vi "DCMotorControl_v2.vi"() -> ()   [LabVIEW 2019]
uses:
  <vilib>/myRIO/Common/Instrument Driver Framework/myRIO v1.0/Encoder/typedefs/Encoder Signal Mode.ctl
  <vilib>/myRIO/Instrument Drivers/Onboard IO/Encoder/typedefs/Encoder Reference.ctl
  <vilib>/myRIO/Common/Instrument Driver Framework/Utilities/typedefs/myRIO Generic Hardware Reference.ctl
  <vilib>/myRIO/Common/Instrument Driver Framework/Utilities/typedefs/Hardware Version Enum.ctl
  <vilib>/myRIO/Common/Instrument Driver Framework/Utilities/typedefs/myRIO v1.0 Reference.ctl
  <vilib>/myRIO/Common/Instrument Driver Framework/Utilities/typedefs/Generic FPGA Reference.ctl
  <vilib>/myRIO/Common/Instrument Driver Framework/myRIO v1.0/Encoder/typedefs/Encoder Channels Enum.ctl
  <vilib>/myRIO/Common/Instrument Driver Framework/myRIO v1.0/Encoder/typedefs/Encoder Configuration v1.0.ctl
  <vilib>/userDefined/High Color/nirio_resource_hc.ctl
  <vilib>/Platform/TimedLoop/XDataNode/timing_clust.ctl
  <vilib>/Platform/TimedLoop/XDataNode/nitl_modes.ctl
  <vilib>/Platform/TimedLoop/XDataNode/wakeup.ctl
  <vilib>/myRIO/Instrument Drivers/Onboard IO/DIO/typedefs/DIO Reference.ctl
  <vilib>/myRIO/Common/Instrument Driver Framework/myRIO v1.0/DIO/typedefs/DIO Channels List.ctl
  <vilib>/myRIO/Common/Instrument Driver Framework/myRIO v1.0/DIO/typedefs/DIO Channels Enum.ctl
  <vilib>/myRIO/Instrument Drivers/Onboard IO/PWM/typedefs/PWM Reference.ctl
  <vilib>/myRIO/Common/Instrument Driver Framework/myRIO v1.0/PWM/typedefs/PWM Channels Enum.ctl
  <vilib>/myRIO/Instrument Drivers/Onboard IO/PWM/typedefs/PWM Configuration.ctl
  <vilib>/myRIO/Common/Instrument Driver Framework/Utilities/vis/Is FPGA Ref Available.vi
  <vilib>/myRIO/Common/Instrument Driver Framework/myRIO v1.0/Encoder/vis/myRIO v1.1 Open Encoder.vi
  <vilib>/myRIO/Instrument Drivers/Onboard IO/Encoder/vis/Read.vi
  <vilib>/myRIO/Common/Instrument Driver Framework/myRIO v1.0/DIO/vis/myRIO v1.1 Open DIO.vi
  <vilib>/myRIO/Instrument Drivers/Onboard IO/DIO/vis/Write.vi
  <vilib>/myRIO/Common/Instrument Driver Framework/myRIO v1.0/PWM/vis/myRIO v1.1 Open PWM.vi
  <vilib>/myRIO/Instrument Drivers/Onboard IO/PWM/vis/Set Duty Cycle and Frequency.vi
  <vilib>/myRIO/Common/Instrument Driver Framework/Utilities/vis/Validate Channels.vi
  <vilib>/myRIO/Common/Instrument Driver Framework/myRIO v1.0/Encoder/vis/myRIO v1.0 Reserve Encoder.vi
  <vilib>/myRIO/Common/Instrument Driver Framework/myRIO v1.0/DIO/vis/myRIO v1.0 Reserve DIO.vi
  <vilib>/myRIO/Common/Instrument Driver Framework/myRIO v1.0/PWM/vis/myRIO v1.0 Reserve PWM.vi
  <vilib>/myRIO/Common/Instrument Driver Framework/myRIO v1.0/Encoder/vis/myRIO v1.0 Build MUX Configuration Encoder.vi
  <vilib>/myRIO/Common/Instrument Driver Framework/myRIO v1.0/Resource Manager/vis/myRIO v1.0 Reserve Channel List.vi
  <vilib>/myRIO/Common/Instrument Driver Framework/myRIO v1.0/DIO/vis/myRIO v1.0 Build MUX Configuration DIO.vi
  <vilib>/myRIO/Common/Instrument Driver Framework/myRIO v1.0/PWM/vis/myRIO v1.0 Build MUX Configuration PWM.vi
  <vilib>/myRIO/Common/Instrument Driver Framework/myRIO v1.0/Resource Manager/vis/myRIO v1.0 Create Configuration List.vi
  <vilib>/myRIO/Common/Instrument Driver Framework/myRIO v1.0/Resource Manager/vis/myRIO v1.0 Reserve Channel.vi
  <vilib>/myRIO/Common/Instrument Driver Framework/myRIO v1.0/Resource Manager/vis/myRIO v1.0 Unreserve Channel.vi
  <vilib>/myRIO/Common/Instrument Driver Framework/myRIO v1.0/Resource Manager/vis/myRIO v1.0 Build Mutex Name.vi
  <vilib>/Utility/VariantDataType/GetNumericInfo.vi
  <vilib>/Utility/error.llb/Error Cluster From Error Code.vi
  <vilib>/myRIO/Common/Instrument Driver Framework/myRIO v1.0/myRIO v1.1 Open.vi
  <vilib>/myRIO/Common/Instrument Driver Framework/Utilities/vis/IO Manager.vi
  <vilib>/myRIO/Common/Instrument Driver Framework/Utilities/vis/Configuration Manager.vi
  <vilib>/myRIO/Common/Instrument Driver Framework/myRIO v1.0/Resource Manager/vis/myRIO v1.0 Configure IO.vi
  <vilib>/myRIO/Common/Instrument Driver Framework/myRIO v1.0/myRIO v1.0 Close.vi
  <vilib>/myRIO/Common/Instrument Driver Framework/myRIO v1.0/Encoder/vis/myRIO v1.0 Configure Encoder.vi
  <vilib>/myRIO/Common/Instrument Driver Framework/myRIO v1.0/Encoder/vis/myRIO v1.0 Read Encoder.vi
  <vilib>/myRIO/Common/Instrument Driver Framework/myRIO v1.0/DIO/vis/myRIO v1.0 Write DIO.vi
  <vilib>/myRIO/Common/Instrument Driver Framework/myRIO v1.0/PWM/vis/myRIO v1.0 Write PWM.vi
  <vilib>/Utility/file.llb/Write Delimited Spreadsheet (DBL).vi
  <vilib>/myRIO/Express VI/Onboard IO/Encoder/Encoder Express VI.xnode
  <vilib>/myRIO/Instrument Drivers/Onboard IO/Encoder/vis/myRIO Encoder Open.xnode
  <vilib>/myRIO/Common/Instrument Driver Framework/myRIO v1.0/Encoder/typedefs/Encoder Count Direction Enum.ctl
  <vilib>/Platform/TimedLoop/XDataNode/XDataNode.xnode
  <vilib>/myRIO/Express VI/Onboard IO/DO/DO Express VI.xnode
  <vilib>/myRIO/Instrument Drivers/Onboard IO/DIO/vis/myRIO DIO Open.xnode
  <vilib>/myRIO/Express VI/Onboard IO/PWM/PWM Express VI.xnode
  <vilib>/myRIO/Instrument Drivers/Onboard IO/PWM/vis/myRIO PWM Open.xnode
  <vilib>/myRIO/Instrument Drivers/Onboard IO/Encoder/Encoder.lvlib
  <vilib>/Platform/TimedLoop/XDataNode/XDNodeRunTimeDep.lvlib
  <vilib>/myRIO/Instrument Drivers/Onboard IO/PWM/PWM.lvlib
  <vilib>/myRIO/Instrument Drivers/Onboard IO/DIO/DIO.lvlib
panel:
  out "Velocity Graph":cluster{dbl[], dbl[]}[](graph)
  out "Position Graph":cluster{dbl[], dbl[]}[](graph)
  in  "plot freq.":i32=100
  in  "format (%.3f)":string="%.3f"
  in  "file path (dialog if empty)":path
  in  "data of 5th order formula\nts,tair,a1-a6":dbl[](array[numeric])=[0.163616269216122, 0.27489641502463, 771965.39318528, -201617.027694185, 8828.08396944145, -2683.04589908678, 1085.57303422127, -48.5860395324432]
  in  "first or second tripod":bool=TRUE
  in  "buffer ratio":dbl=0.3
  in  "T_ratio":dbl=10.0
  in  "t_shift":dbl=0.000125
  in  "Encoder_Count":dbl=54991.0
  out "Counter Value":i32
  out "encoder_position":dbl
  in  "Gain":T1={"P Gain"=0.5, "I Gain"=0.0, "D Gain"=0.005}
  in  "Frequency [Hz]":dbl=1000.0
  in  "stop":bool
  out "Duty":dbl
  out "Position(deg)":cluster{dbl, dbl}(graph)
  out "Velocity(deg/s)":cluster{"set point":dbl, dbl}(graph)
  out "Time":dbl
  out "Duty cycle":dbl(graph)
  in  "Loop Period":i64=5
  # "v = 1; a = 15"
  # "v = 1.25; a = 15"
  # "v = 1.5; a = 15"
  # "0.184067181524967\n0.263820978418769\n256152.551336786\n-30272.30000274\n-9876.03760433421\n-1096.38594197941\n885.91817900106\n-44.6781799901984"
  # "0.215241998794118\n0.254514142390288\n4771.41078363533\n62185.8763006578\n-22508.5336527453\n390.805502041188\n686.695311017595\n-40.4128145310291"
  # "0.163616269216122\n0.27489641502463\n771965.39318528\n-201617.027694185\n8828.08396944145\n-2683.04589908678\n1085.57303422127\n-48.5860395324432"
  # "v = 1.75; a = 15"
  # "v = 2; a = 15"
  # "v = 2.25; a = 15"
  # "0.148651048423414\n0.288542414074344\n1776973.44893281\n-511591.467559457\n38775.9830765103\n-4576.94506688942\n1289.39828252671\n-52.3115561007577"
  # "0.136976185169818\n0.304016701267508\n3461279.85083822\n-993110.73746345\n80544.6579529191\n-6699.48295844177\n1494.82265451498\n-55.8934424469099"
  # "0.134381902205816\n0.369022171779704\n3272804.8365432\n-899365.569589567\n71225.2463409934\n-7039.10791102172\n1512.66147498591\n-59.3408899720725"
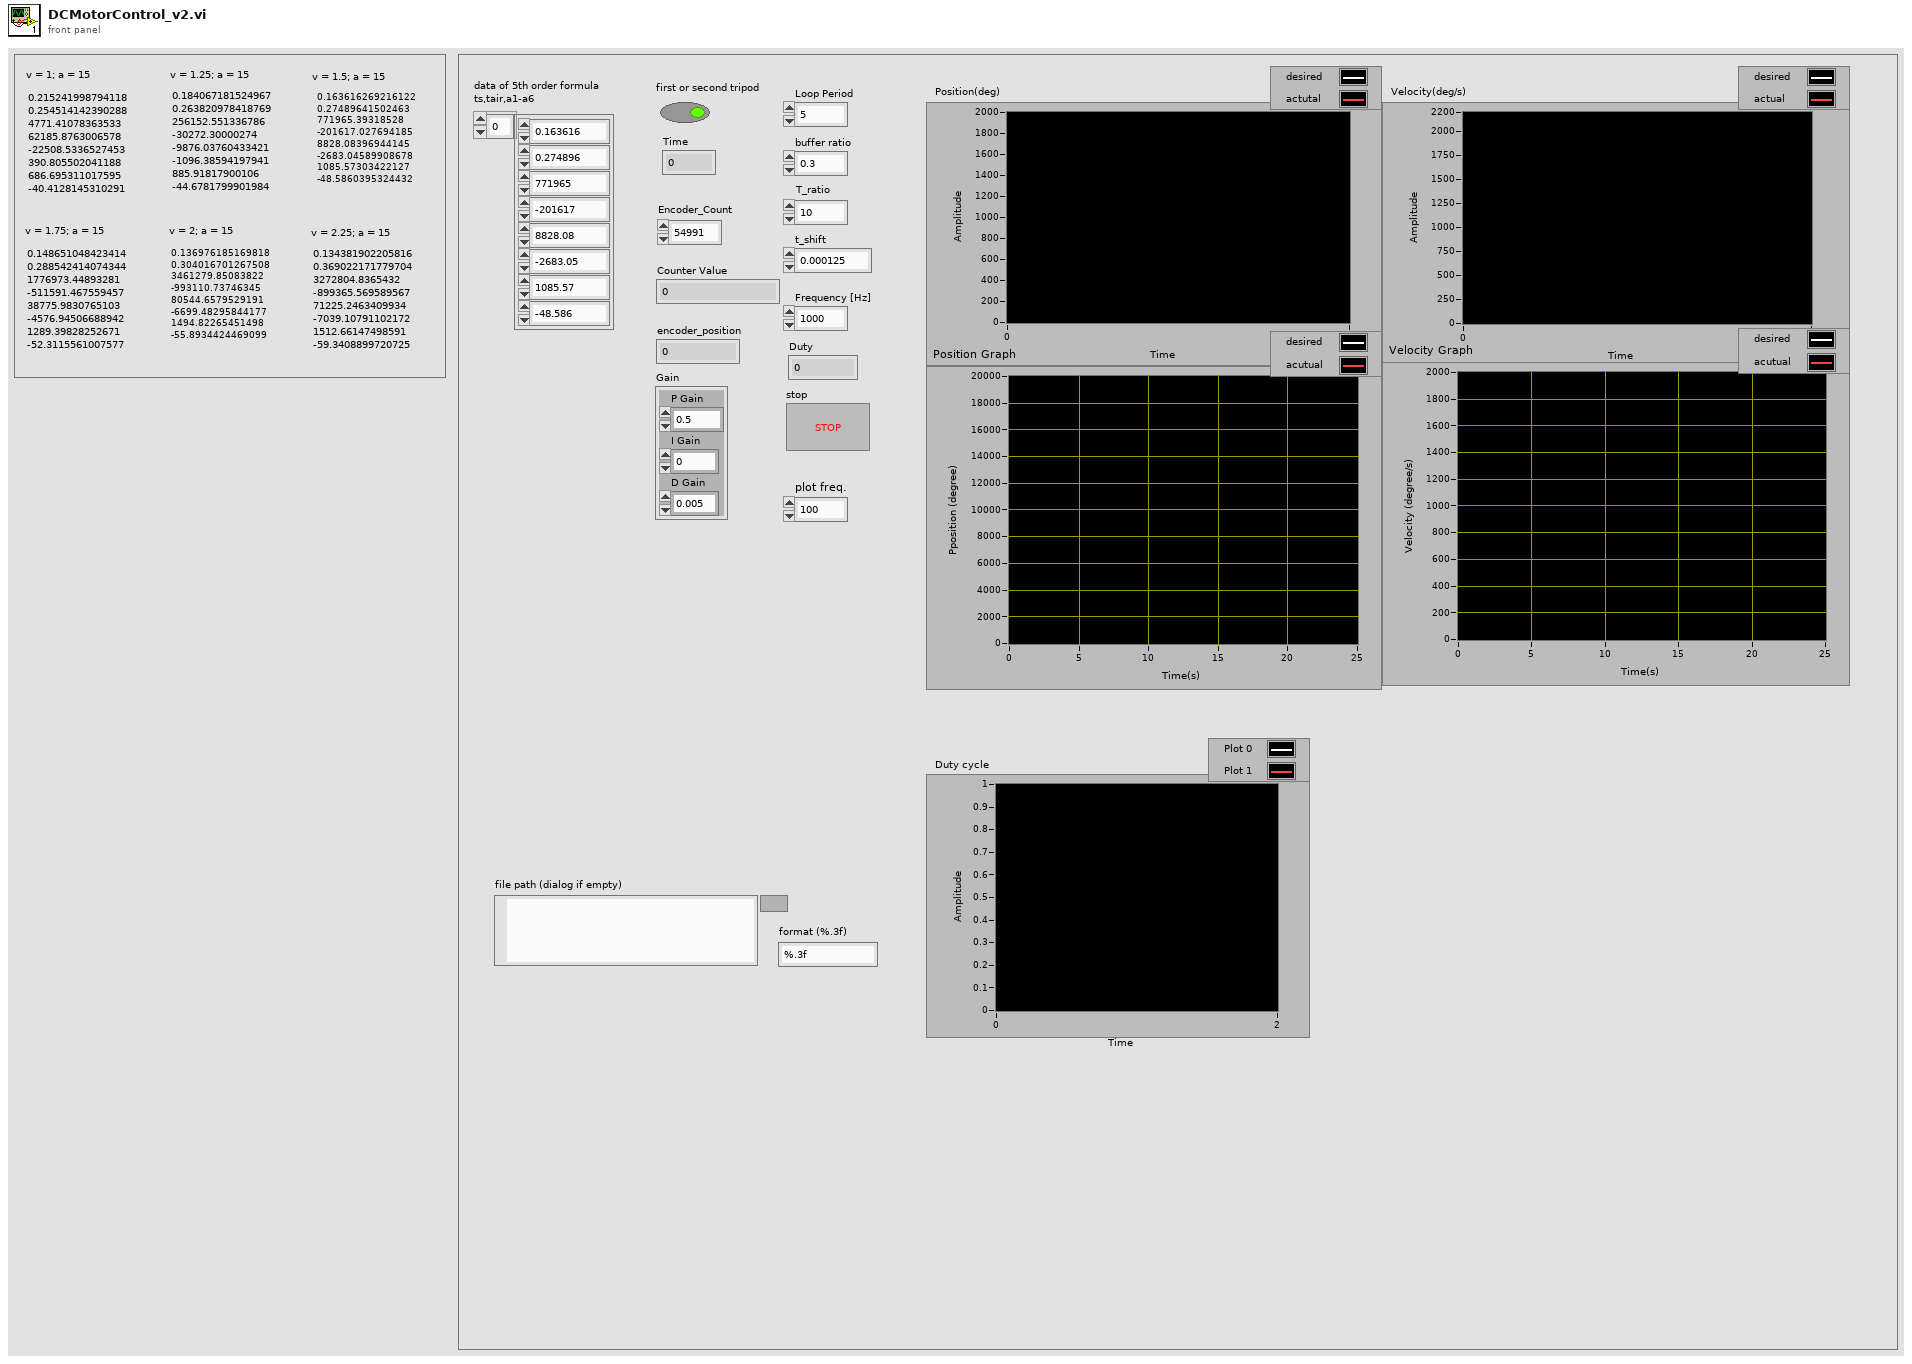
[diagram p1: front panel]
types:
  T1 = cluster{"P Gain":dbl, "I Gain":dbl, "D Gain":dbl}
  T2 = typedef "Encoder.lvlib/Encoder Reference.ctl" = cluster{"myRIO Reference":T3, "Encoder Channels Enum":T7}
  T3 = typedef "myRIO Generic Hardware Reference.ctl" = cluster{"myRIO Model":T4, "myRIO Hardware Reference":T5}
  T4 = typedef "Hardware Version Enum.ctl" = enum16{"Unknown", "myRIO-1900", "myRIO-1950", "roboRIO", "NI ELVIS RIO CM", "ELVIS III"}
  T5 = typedef "myRIO v1.0 Reference.ctl" = cluster{"Generic FPGA Reference":T6, "Allow multiple opens":bool}
  T6 = typedef "Generic FPGA Reference.ctl" = refnum<k20>
  T7 = typedef "Encoder Channels Enum.ctl" = enum16{"Not Connected", "C/ENC0", "C/ENC1", "A/ENC", "A/ENC0", "A/ENC1", "A/ENC2", "A/ENC3", "A/ENC4", "A/ENC5", "A/ENC6", "A/ENC7", "A/ENC8", "A/ENC9", "B/ENC", "B/ENC0", "B/ENC1", "B/ENC2", "B/ENC3", "B/ENC4", "B/ENC5", "B/ENC6", "B/ENC7", "B/ENC8", "B/ENC9", "DIO/ENC0", "DIO/ENC1", "DIO/ENC2", "DIO/ENC3", "DIO/ENC4"}
  T8 = typedef "Encoder Signal Mode.ctl" = enum16{"Quadrature phase signal", "Step and direction signal"}
  T9 = typedef "nirio_resource_hc.ctl" = tag
  T10 = cluster{"set position":dbl, "set position":dbl, "set position":dbl, "set position":dbl, "set position":dbl, "set position":dbl}
  T11 = typedef "DIO.lvlib/DIO Reference.ctl" = cluster{"myRIO Reference":T3, "DIO Channels List":T12}
  T12 = typedef "DIO Channels List.ctl" = T13[]
  T13 = typedef "DIO Channels Enum.ctl" = enum16{"Not Connected", "C/DIO0", "C/DIO1", "C/DIO2", "C/DIO3", "C/DIO4", "C/DIO5", "C/DIO6", "C/DIO7", "A/DIO0", "A/DIO1", "A/DIO2", "A/DIO3", "A/DIO4", "A/DIO5", "A/DIO6", "A/DIO7", "A/DIO8", "A/DIO9", "A/DIO10", "A/DIO11", "A/DIO12", "A/DIO13", "A/DIO14", "A/DIO15", "A/DIO16", "A/DIO17", "A/DIO18", "A/DIO19", "B/DIO0", "B/DIO1", "B/DIO2", "B/DIO3", "B/DIO4", "B/DIO5", "B/DIO6", "B/DIO7", "B/DIO8", "B/DIO9", "B/DIO10", "B/DIO11", "B/DIO12", "B/DIO13", "B/DIO14", "B/DIO15", "B/DIO16", "B/DIO17", "B/DIO18", "B/DIO19", "LED0", "LED1", "LED2", "LED3", "Button0", "DIO/DIO0", "DIO/DIO1", "DIO/DIO2", "DIO/DIO3", "DIO/DIO4", "DIO/DIO5", "DIO/DIO6", "DIO/DIO7", "DIO/DIO8", "DIO/DIO9", "SPI/CS0", "SPI/CS1", "SPI/CS2", "SPI/CS3", "LED RADIO (Green)", "LED RADIO (Red)", "LED COMM (Green)", "LED COMM (Red)", "LED MODE (Green)", "LED MODE (Red)"}
  T14 = typedef "PWM.lvlib/PWM Reference.ctl" = cluster{"myRIO Reference":T3, "PWM Channels Enum":T15, "PWM Configuration":T16}
  T15 = typedef "PWM Channels Enum.ctl" = enum16{"Not Connected", "C/PWM0", "C/PWM1", "A/PWM0", "A/PWM1", "A/PWM2", "A/PWM3", "A/PWM4", "A/PWM5", "A/PWM6", "A/PWM7", "A/PWM8", "A/PWM9", "A/PWM10", "A/PWM11", "A/PWM12", "A/PWM13", "A/PWM14", "A/PWM15", "A/PWM16", "A/PWM17", "A/PWM18", "A/PWM19", "B/PWM0", "B/PWM1", "B/PWM2", "B/PWM3", "B/PWM4", "B/PWM5", "B/PWM6", "B/PWM7", "B/PWM8", "B/PWM9", "B/PWM10", "B/PWM11", "B/PWM12", "B/PWM13", "B/PWM14", "B/PWM15", "B/PWM16", "B/PWM17", "B/PWM18", "B/PWM19", "PWM/PWM0", "PWM/PWM1", "PWM/PWM2", "PWM/PWM3", "PWM/PWM4", "PWM/PWM5", "PWM/PWM6", "PWM/PWM7", "PWM/PWM8", "PWM/PWM9"}
  T16 = typedef "PWM.lvlib/PWM Configuration.ctl" = cluster{"Frequency":dbl, "Duty Cycle":dbl}
  T17 = typedef "XDNodeRunTimeDep.lvlib/timing_clust.ctl" = cluster{"Expected End [f-1]":u64, "Actual End [f-1]":u64, "Finished Late? [f-1]":bool, "Expected End [i-1]":u64, "Actual End [i-1]":u64, "Finished Late? [i-1]":bool, "Expected Start [i]":u64, "Actual Start [i]":u64, "Expected Start [f]":u64, "Actual Start [f]":u64, "Source Name":string, "Structure Name":string, "Period":i64, "Deadline":i64, "Offset":i64, "Start":i64, "Priority":i32, "Timeout":i32, "Mode":T18, "Wakeup Reason":T19, "Error":errorcluster, "Source Type":string, "Secondary Source Type":string, "Global End Time":u64, "Global Start Time":u64, "Frame Duration":u64, "Iteration Duration":u64, "Assigned CPU":i32, "I/O Scan Engine Mode":u32}
  T18 = typedef "XDNodeRunTimeDep.lvlib/nitl_modes.ctl" = enum32{"No Change", "Process missed periods, maintain original phase", "Discard missed periods, maintain original phase", "Process missed periods, ignore original phase", "Discard missed periods, ignore original phase"}
  T19 = typedef "XDNodeRunTimeDep.lvlib/wakeup.ctl" = enum32{"Normal", "Aborted", "Asynchronous wakeup", "Timing source error", "Timed loop error", "Timeout"}
  T20 = cluster{"[0]":dbl, "[1]":dbl, "[2]":dbl, "[3]":dbl, "[4]":dbl, "[5]":dbl}
  T21 = cluster{"set position":i32, "set position":i32, "set position":i32, "set position":i32, "set position":i32, "set position":i32}
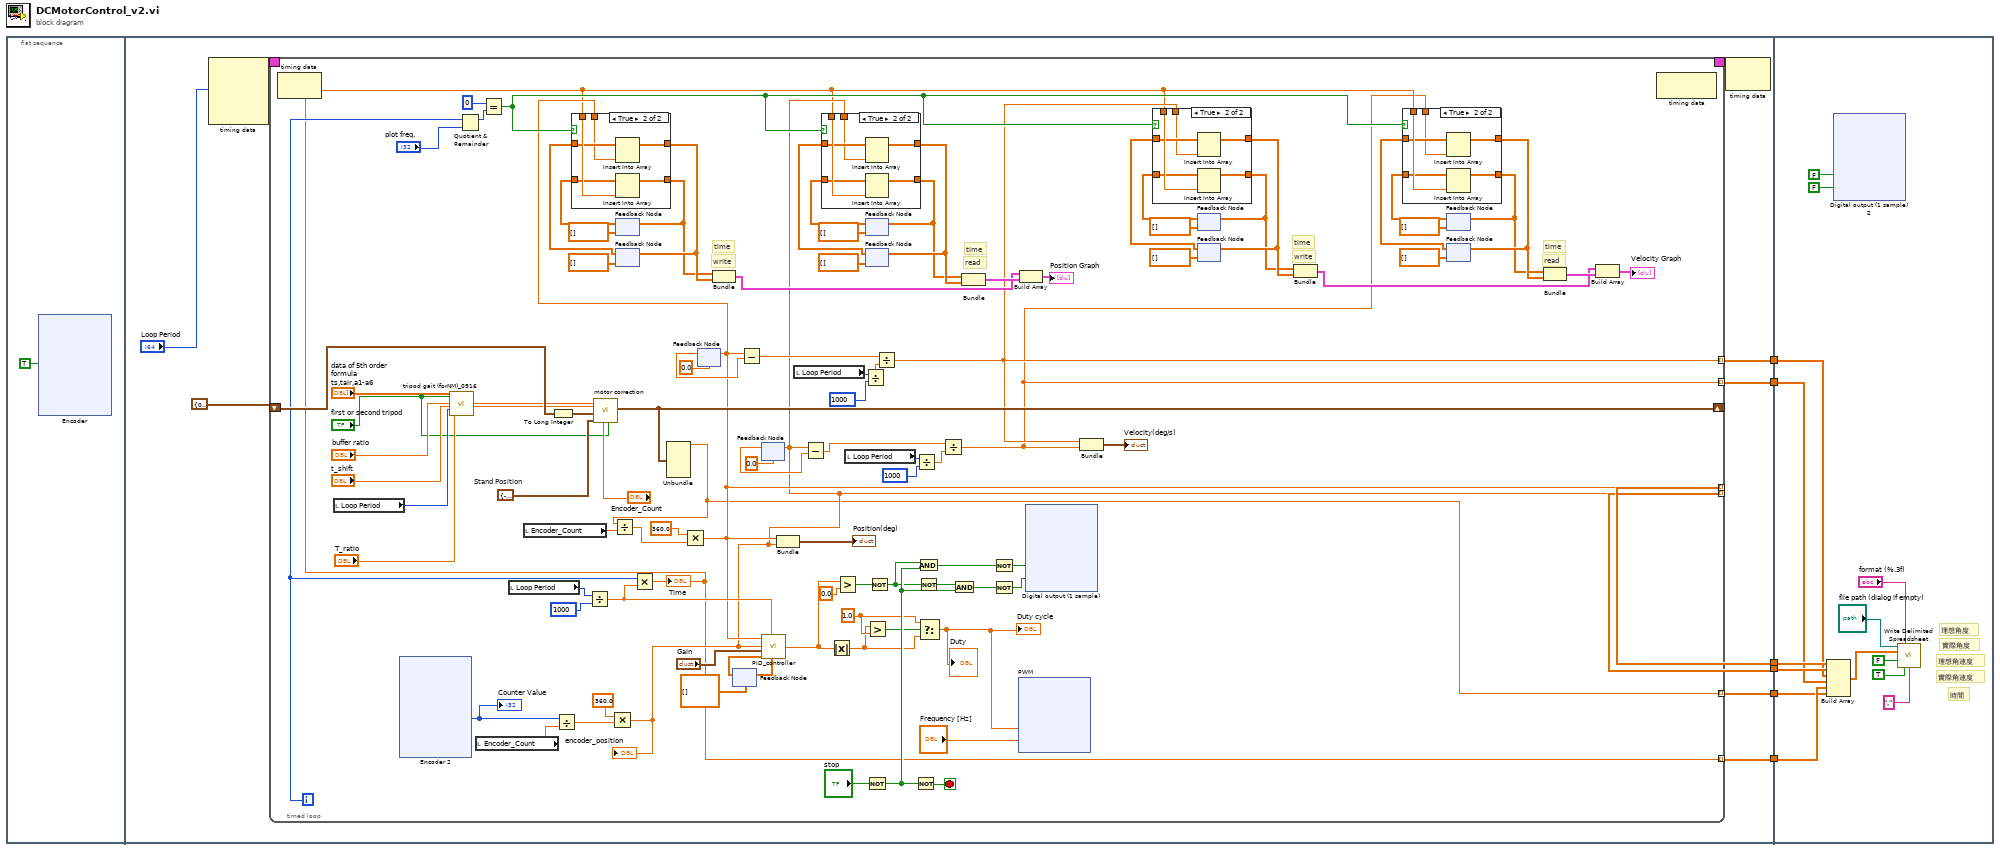
[diagram p0: block diagram]
diagram:
  n1 = flat-sequence {
    tunnel: [w59] -> w6
    tunnel: [w58] -> w5
    tunnel: [w57] -> w4
    tunnel: [w56] -> w3
    tunnel: [w55] -> w2
    tunnel: [w54] -> w1
    tunnel: w6 -> [w328]
    tunnel: w5 -> [w327]
    tunnel: w4 -> [w326]
    tunnel: w3 -> [w325]
    tunnel: w2 -> [w319]
    tunnel: w1 -> [w318]
    frame #0 {
      n2 = xnode "Encoder"("Reset Counter"=TRUE) -> ()  [unwired: 1 in, 4 out]
    }
    frame #1 {
      n3 = node-c288("Loop Period") -> (w63:T17)  [unwired: 3 in]
      n4 = timed-loop {
        timing: w63 -> [_]
        timing-out: [_] -> w62
        shift-right: [w154] -> _
        shift-left: T10 {"set position"=0.0, "set position"=0.0, "set position"=0.0, "set position"=0.0, "set position"=0.0, "set position"=0.0} ("Setpoint_to_motor") -> [w152]
        tunnel: [w68] -> w58 mode=indexing
        tunnel: [w69] -> w59 mode=indexing
        tunnel: [w65] -> w56 mode=indexing
        tunnel: [w67] -> w57 mode=indexing
        tunnel: [w66] -> w55 mode=indexing
        tunnel: [w64] -> w54 mode=indexing
        i -> [w96]
        stop <- w131 stop-if-true
        w139 = 1.0 ("y")
        w151 = T20 {"[0]"=-27495.5, "[1]"=-27495.5, "[2]"=-27495.5, "[3]"=-27495.5, "[4]"=-27495.5, "[5]"=-27495.5}  # Stand Position
        # "time"
        # "read"
        # "time"
        # "write"
        # "time"
        # "read"
        # "time"
        # "write"
        n5 = node-c288() -> ()  [unwired: 1 in, 1 out]
        n6 = local read "Loop Period"() -> (w158:i64)
        n7 = xnode "Encoder 2"() -> ("Counter Value"=w106:i32)  [unwired: 2 in, 3 out]
        "Counter Value" <- w106
        n8 = call "tripod gait (forNM)_0916.vi"("data of 5th order formula\nts,tair,a1-a6"="data of 5th order formula\nts,tair,a1-a6", "first or second"="first or second tripod", "buffer ratio"="buffer ratio", "t_shift"="t_shift", "sample time"=w158, "T_ratio"="T_ratio") -> ("Set Point"=w114:dbl, "Set Point 2"=w113:dbl)  [unwired: 4 in, 16 out]
        n9 = Quotient & Remainder(x=w96, y="plot freq.") -> (x-y*floor(x/y)=w70:i32)  [unwired: 1 out]
        n10 = local read "Encoder_Count"() -> (w155:dbl)
        n11 = Equal?(x=0, y=w70) -> (x = y?=w71:bool)
        n12 = local read "Loop Period"() -> (w122:i64)
        n13 = local read "Encoder_Count"() -> (w120:dbl)
        n14 = To Long Integer(number=w152) -> (32bit integer=w153:T21)
        n15 = Divide(x=w106, y=w155) -> (x/y=w115:dbl)
        n16 = Divide(x=w122, y=i64 1000) -> (x/y=w111:dbl)
        n17 = call "motor correction.vi"("first or second"="first or second tripod", "Encoder_Count"="Encoder_Count", "Stand Position"=w151, "encoder position"=w153, "set position 2"=w113, "set position"=w114) -> ("Setpoint_to_motor"=w154:T10)  [unwired: 4 in, 1 out]
        n18 = Multiply(x=360.0, y=w115) -> (x*y=w68:dbl)
        "encoder_position" <- w68
        n19 = feedback #1(dbl[] []) -> (w104:dbl[])
        n20 = feedback #2(dbl[] []) -> (w101:dbl[])
        n21 = Multiply(x=w96, y=w111) -> (x*y=w66:dbl)
        "Time" <- w66
        n22 = Unbundle(w154) -> ("set position"=w64:dbl)  [unwired: 5 out]
        n23 = Divide(x=w64, y=w120) -> (x/y=w118:dbl)
        n24 = Multiply(x=360.0, y=w118) -> (x*y=w69:dbl)
        n25 = case shown="True" w71 {
          tunnel: w69 -> [_ w189]
          tunnel: w66 -> [_ w194]
          tunnel: [w188 w193] -> w98
          tunnel: w104 -> [w188 w192]
          tunnel: [w187 w191] -> w99
          tunnel: w101 -> [w187 w190]
          frame False {
          }
          frame True {
            n26 = Insert Into Array(array=w190, new element=w189) -> (w191:dbl[])  [unwired: 1 in]
            n27 = Insert Into Array(array=w192, new element=w194) -> (w193:dbl[])  [unwired: 1 in]
          }
        }
        n28 = feedback-in #1(w98) -> ()
        n29 = feedback-in #2(w99) -> ()
        n30 = feedback #3(0.0) -> (w126:dbl)
        n31 = feedback-in #3(w69) -> ()
        n32 = Bundle(w98, w99) -> (w87:cluster{dbl[], dbl[]})  [unwired: 1 in]
        n33 = feedback #4(dbl[] [] ("state(k)")) -> (w150:dbl[])
        n34 = Subtract(x=w69, y=w126) -> (x-y=w109:dbl)
        n35 = feedback #5(0.0) -> (w108:dbl)
        n36 = feedback-in #5(w68) -> ()
        n37 = call "PID_controller.vi"("Time Period"=w111, "state(k-1)"=w150, "Gain"="Gain", "variable"=w68, "set point"=w69) -> ("PID gain"=w132:dbl, "state(k)"=w149:dbl[])
        n38 = feedback-in #4(w149) -> ()
        n39 = Bundle(w69, w68) -> (→"Position(deg)":cluster{dbl, dbl})  [unwired: 1 in]
        n40 = local read "Loop Period"() -> (w125:i64)
        n41 = Subtract(x=w68, y=w108) -> (x-y=w110:dbl)
        n42 = Absolute Value(x=w132) -> (abs(x)=w138:dbl)
        n43 = Greater?(x=w132, y=0.0) -> (0:w141:bool)
        n44 = local read "Loop Period"() -> (w129:i64)
        n45 = Divide(x=w125, y=i64 1000) -> (x/y=w124:dbl)
        n46 = feedback #6(dbl[] []) -> (w94:dbl[])
        n47 = feedback #7(dbl[] []) -> (w91:dbl[])
        n48 = case shown="True" w71 {
          tunnel: w68 -> [_ w181]
          tunnel: w66 -> [_ w186]
          tunnel: [w180 w185] -> w89
          tunnel: w94 -> [w180 w184]
          tunnel: [w179 w183] -> w90
          tunnel: w91 -> [w179 w182]
          frame False {
          }
          frame True {
            n49 = Insert Into Array(array=w182, new element=w181) -> (w183:dbl[])  [unwired: 1 in]
            n50 = Insert Into Array(array=w184, new element=w186) -> (w185:dbl[])  [unwired: 1 in]
          }
        }
        n51 = feedback-in #6(w89) -> ()
        n52 = feedback-in #7(w90) -> ()
        n53 = Not(x="stop") -> (.not. x?=w143:bool)
        n54 = Greater?(x=w138, y=w139) -> (0:w140:bool)
        n55 = Not(x=w141) -> (.not. x?=w137:bool)
        n56 = Divide(x=w109, y=w124) -> (x/y=w67:dbl)
        n57 = Not(x=w143) -> (.not. x?=w131:bool)
        n58 = Divide(x=w129, y=i64 1000) -> (x/y=w127:dbl)
        n59 = And(x=w137, y=w143) -> (x .and. y?=w134:bool)
        n60 = Not(x=w137) -> (.not. x?=w145:bool)
        n61 = Select(t=w139, s=w140, f=w138) -> (s? t:f=w105:dbl)
        "Duty" <- w105
        "Duty cycle" <- w105
        n62 = Divide(x=w110, y=w127) -> (x/y=w65:dbl)
        n63 = And(x=w145, y=w143) -> (x .and. y?=w136:bool)
        n64 = Bundle(w89, w90) -> (w88:cluster{dbl[], dbl[]})  [unwired: 1 in]
        n65 = Not(x=w134) -> (.not. x?=w133:bool)
        n66 = Not(x=w136) -> (.not. x?=w135:bool)
        n67 = xnode "PWM"("Duty Cycle"=w105, "Frequency [Hz]"="Frequency [Hz]") -> ()  [unwired: 1 in, 1 out]
        n68 = Build Array(w87, w88) -> (→"Position Graph":cluster{dbl[], dbl[]}[])
        n69 = xnode "Digital output (1 sample)"("A/DIO0 (Pin 11)"=w133, "A/DIO1 (Pin 13)"=w135) -> ()  [unwired: 1 in, 1 out]
        n70 = Bundle(w67, w65) -> (→"Velocity(deg/s)":cluster{dbl, dbl})  [unwired: 1 in]
        n71 = feedback #8(dbl[] []) -> (w86:dbl[])
        n72 = feedback #9(dbl[] []) -> (w83:dbl[])
        n73 = case shown="True" w71 {
          tunnel: w67 -> [_ w173]
          tunnel: w66 -> [_ w178]
          tunnel: [w172 w177] -> w81
          tunnel: w86 -> [w172 w176]
          tunnel: [w171 w175] -> w82
          tunnel: w83 -> [w171 w174]
          frame False {
          }
          frame True {
            n74 = Insert Into Array(array=w174, new element=w173) -> (w175:dbl[])  [unwired: 1 in]
            n75 = Insert Into Array(array=w176, new element=w178) -> (w177:dbl[])  [unwired: 1 in]
          }
        }
        n76 = feedback-in #8(w81) -> ()
        n77 = feedback-in #9(w82) -> ()
        n78 = Bundle(w81, w82) -> (w72:cluster{dbl[], dbl[]})  [unwired: 1 in]
        n79 = feedback #10(dbl[] []) -> (w79:dbl[])
        n80 = feedback #11(dbl[] []) -> (w76:dbl[])
        n81 = case shown="True" w71 {
          tunnel: w65 -> [_ w165]
          tunnel: w66 -> [_ w170]
          tunnel: [w164 w169] -> w74
          tunnel: w79 -> [w164 w168]
          tunnel: [w163 w167] -> w75
          tunnel: w76 -> [w163 w166]
          frame False {
          }
          frame True {
            n82 = Insert Into Array(array=w166, new element=w165) -> (w167:dbl[])  [unwired: 1 in]
            n83 = Insert Into Array(array=w168, new element=w170) -> (w169:dbl[])  [unwired: 1 in]
          }
        }
        n84 = feedback-in #10(w74) -> ()
        n85 = feedback-in #11(w75) -> ()
        n86 = Bundle(w74, w75) -> (w73:cluster{dbl[], dbl[]})  [unwired: 1 in]
        n87 = Build Array(w72, w73) -> (→"Velocity Graph":cluster{dbl[], dbl[]}[])
        n88 = node-c288() -> ()  [unwired: 1 in, 1 out]
      }
      n89 = node-c288(w62) -> ()  [unwired: 1 out]
    }
    frame #2 {
      # "時間"
      # "實際角度"
      # "理想角度"
      # "實際角速度"
      # "理想角速度"
      n90 = Build Array(w328, w327, w326, w325, w319, w318) -> (w324:dbl[][])
      n91 = xnode "Digital output (1 sample) 2"("A/DIO0 (Pin 11)"=FALSE, "A/DIO1 (Pin 13)"=FALSE) -> ()  [unwired: 1 in, 1 out]
      n92 = call-poly <vilib>:"Write Delimited Spreadsheet.vi"("file path (dialog if empty)"="file path (dialog if empty)", "format (%.3f)"="format (%.3f)", "2D data"=w324, "append to file? (new file:F)"=FALSE, "transpose? (no:F)"=TRUE, "delimiter (\\t)"="," ("delimiter (\\t)")) -> ()  [unwired: 8 in, 2 out]
    }
  }
